vi "Set_Max.vi"(0 "VisaCluster":T2, 7 "Max":T1=enum."MAX/MIN", 11 "error in (no error)":errorcluster) -> (4 "VisaCluster":T2, 6 "Max 2":T1=enum."MAX/MIN", 8 "Answer":string, 15 "error out":errorcluster)   [LabVIEW 2014, in "FH 55.lvlib"]
doc: "The VI selects one of three instrument operating modes: \nMax off, \nShow Max,\nShow Min/Max.\n\nDurch das VI kann zwischen den oben gelisteten Ausgaben gewählt werden."
uses:
  FH 55.lvlib
  TypeDef/VisaCluster.ctl
  TypeDef/Max.ctl
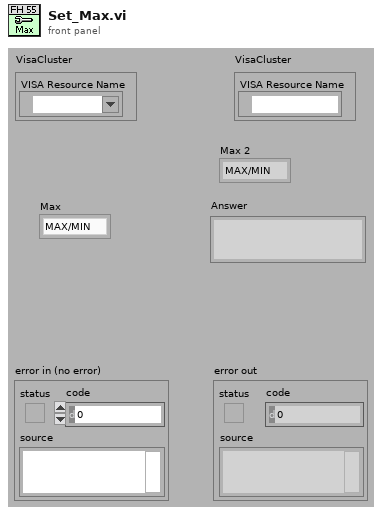
[diagram p1: front panel]
types:
  T1 = typedef "FH 55.lvlib/Max.ctl" = enum16{"MAX off", "Show MAX", "MAX/MIN"}
  T2 = typedef "FH 55.lvlib/VisaCluster.ctl" = cluster{"VISA Resource Name":refnum<visa-resource-name>}
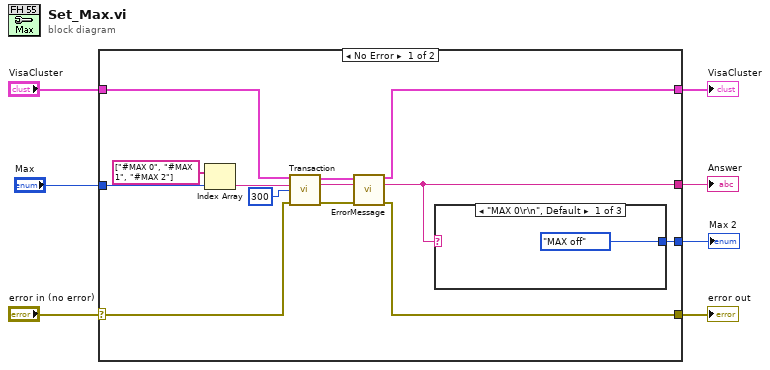
[diagram p0: block diagram]
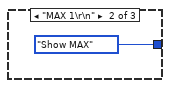
[diagram p2: hidden frame]
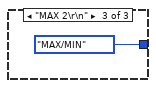
[diagram p3: hidden frame]
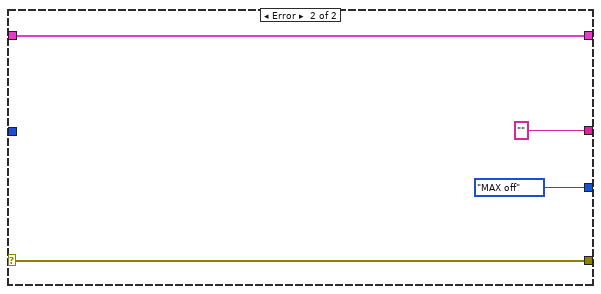
[diagram p4: hidden frame]
diagram:
  n1 = case shown="No Error" "error in (no error)" {
    selector: "error in (no error)" -> [w19 w26]
    tunnel: "VisaCluster" -> [w20 w27]
    tunnel: "Max" -> [w15 _]
    tunnel: [w11 w27] -> w3
    tunnel: [w10 w26] -> w5
    tunnel: [w9 ""] -> w4
    tunnel: [w8 Max."MAX off" ("Max 2")] -> w1
    frame No Error {
      n2 = Index Array(array=string[] ["#MAX 0", "#MAX 1", "#MAX 2"], index=w15) -> (element=w13:string)
      n3 = call "Transaction.vi"("VisaCluster"=w20, "Command"=w13, "Time (150) ms"=u32 300, "error in (no error)"=w19) -> ("VisaCluster"=w16:T2, "Answer"=w17:string, "error out"=w18:errorcluster)  [unwired: 8 in, 1 out]
      n4 = call "ErrorMessage.vi"("VisaCluster"=w16, "Message In"=w17, "error in (no error)"=w18) -> ("VisaCluster"=w11:T2, "Message Out"=w9:string, "error out"=w10:errorcluster)  [unwired: 10 in]
      n5 = case shown="\"MAX 0\\r\\n\", Default" w9 {
        tunnel: [Max."MAX off" ("Max") Max."Show MAX" ("Max") Max."MAX/MIN" ("Max")] -> w8
        frame "MAX 0\r\n", Default {
        }
        frame "MAX 1\r\n" {
        }
        frame "MAX 2\r\n" {
        }
      }
    }
    frame Error {
    }
  }
  "error out" <- w5
  "Answer" <- w4
  "VisaCluster" <- w3
  "Max 2" <- w1
